vi "getError.vi"(8 "error in (no error)":errorcluster, 10 "errorCode":i32, 11 "ElectrometerError in":refnum<class "ElectrometerError.lvclass">) -> (0 "error out":errorcluster, 2 "Error":T1, 3 "ElectrometerError out":refnum<class "ElectrometerError.lvclass">)   [LabVIEW 2016, in "ElectrometerError.lvclass"]
uses:
  ElectrometerError.lvclass
  Controls/errorType.ctl
  ElectrometerError.lvclass/ElectrometerError.ctl
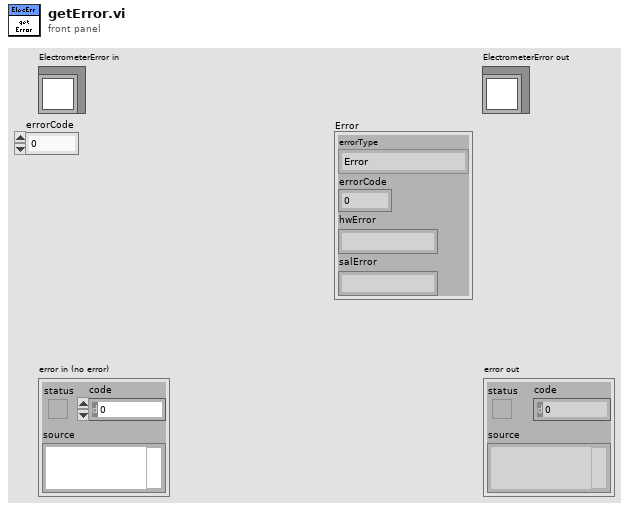
[diagram p1: front panel]
types:
  T1 = typedef "ElectrometerError.lvclass/errorType.ctl" = cluster{"errorType":enum16{"Error", "Warning", "None"}, "errorCode":dbl, "hwError":string, "salError":string}
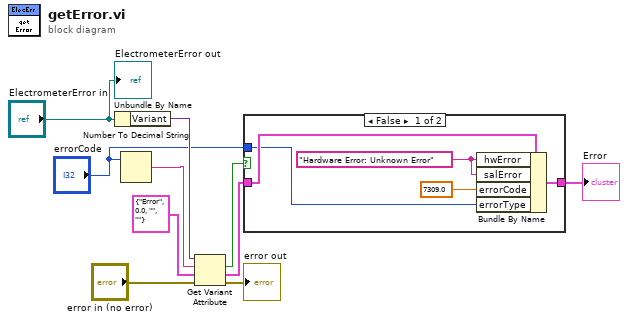
[diagram p0: block diagram]
diagram:
  n1 = Unbundle By Name("ElectrometerError in") -> ("Variant"=w9:variant)
  n2 = Number To Decimal String(number="errorCode") -> (decimal integer string=w1:string)  [unwired: 1 in]
  n3 = Get Variant Attribute(Variant=w9, name=w1, default value (empty Variant)=T1 {"errorType"=enum."Error", "errorCode"=0.0, "hwError"="", "salError"=""} ("error"), error in="error in (no error)") -> (found=w5:bool, value=w4:T1, error out=→"error out":errorcluster)  [unwired: 1 out]
  n4 = case shown="False" w5 {
    tunnel: w4 -> [w15 w16]
    tunnel: [w14 w16] -> w3
    tunnel: "errorCode" -> [w11 _]
    frame False {
      w13 = "Hardware Error: Unknown Error" ("salError")
      n5 = Bundle By Name(cluster=w15, "hwError"=w13, "salError"=w13, "errorCode"=7309.0, "errorType"=w11) -> (w14:T1)
    }
    frame True {
    }
  }
  "Error" <- w3
  "ElectrometerError out" <- "ElectrometerError in"
